vi "Initialize.vi"(4 "stop bits (1.0)":u16(ring)=10 items=["1.0"=10, "1.5"=15, "2.0"=20], 6 "parity (none)":enum16{"None", "Odd", "Even", "Mark", "Space"}(ring), 8 "error in (no error)":errorcluster, 9 "data bits (8)":u16=8, 10 "baud rate (9600)":u32=9600, 11 "port":refnum<visa-resource-name>) -> (0 "error out":errorcluster, 3 "MKS MW out":refnum<class "PL MKS MW.lvclass">)   [LabVIEW 2015, in "PL MKS MW.lvclass"]
doc: "Initializes connection to device using specified settings."
uses:
  PL MKS MW.lvclass
  PL MKS MW.lvclass/PL MKS MW.ctl
panel:
  in  "timeout, ms (300)":u32=300
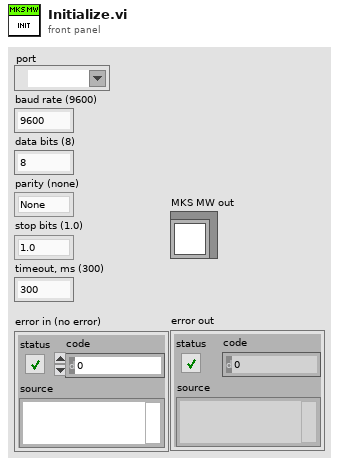
[diagram p1: front panel]
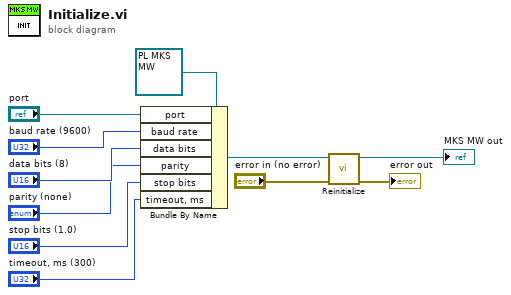
[diagram p0: block diagram]
diagram:
  n1 = Bundle By Name(cluster=refnum<class "PL MKS MW.lvclass"> refnum ("PL Comdel CX.lvclass"), "port"="port", "baud rate"="baud rate (9600)", "data bits"="data bits (8)", "parity"="parity (none)", "stop bits"="stop bits (1.0)", "timeout, ms"="timeout, ms (300)") -> (w11:refnum<class "PL MKS MW.lvclass">)
  n2 = call "Reinitialize.vi"("error in (no error)"="error in (no error)", "MKS MW in"=w11) -> ("error out"=→"error out":errorcluster, "MKS MW out"=→"MKS MW out":refnum<class "PL MKS MW.lvclass">)  [unwired: 8 in]
